vi "CreatePm.vi"(0 "PM_Group in":refnum<class "PM_Group.lvclass">, 5 "error in (no error)":errorcluster, 7 "FPGA API":refnum<class "FPGA API.lvclass">, 9 "ConfigInterface":refnum<class "ConfigInterface.lvclass">, 11 "SV_Publisher":refnum<class "SV_Publisher.lvclass">, 12 "Tags":T1, 13 "Logger":refnum<class "Logger.lvclass">) -> (14 "PM_Group out":refnum<class "PM_Group.lvclass">, 19 "error out":errorcluster)   [LabVIEW 2019, in "PM_Group.lvclass"]
uses:
  PM_Group.lvclass
  C:/Users/H4001/Documents/GitHub/H4000/src/Device_class/Device.lvclass
  C:/Users/H4001/Documents/GitHub/H4000/src/Proccess_class/Proccess.lvclass
  Proccess_class/TAGs.ctl
  FPGA_API_class/FPGA API.lvclass
  ConfigInterface_class/ConfigInterface.lvclass
  SV_Puplisher_class/SV_Publisher.lvclass
  Logger_class/Logger.lvclass
  TypeDef/State PMG.ctl
  PM_Group.lvclass/PM_Group.ctl
  Engine_1DO_2DI_class/DIO.ctl
  FPGA/TypeDef/DO index.ctl
  FPGA/TypeDef/DI index.ctl
  Proccess_class/Proccess.lvclass/Proccess.ctl
  Device_class/Device.lvclass/Device.ctl
  Device_class/Device.lvclass
  Proccess_class/Proccess.lvclass
  Engine_1DO_2DI_class/Engine_1DO_2DI.lvclass
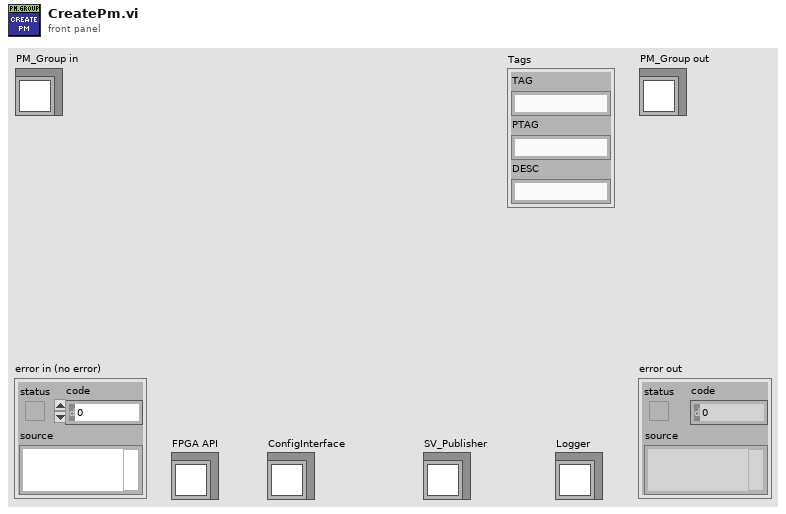
[diagram p1: front panel]
types:
  T1 = typedef "Proccess.lvclass/TAGs.ctl" = cluster{"TAG":string, "PTAG":string, "DESC":string}
  T2 = typedef "State PMG.ctl" = enum16{"NOT READY", "IDLE", "ACTIVE", "ERROR"}
  T3 = typedef "Engine_1DO_2DI.lvclass/DIO.ctl" = cluster{"DO":T4, "DI A":T5, "DI C":T5}
  T4 = typedef "DO index.ctl" = u8
  T5 = typedef "DI index.ctl" = u8
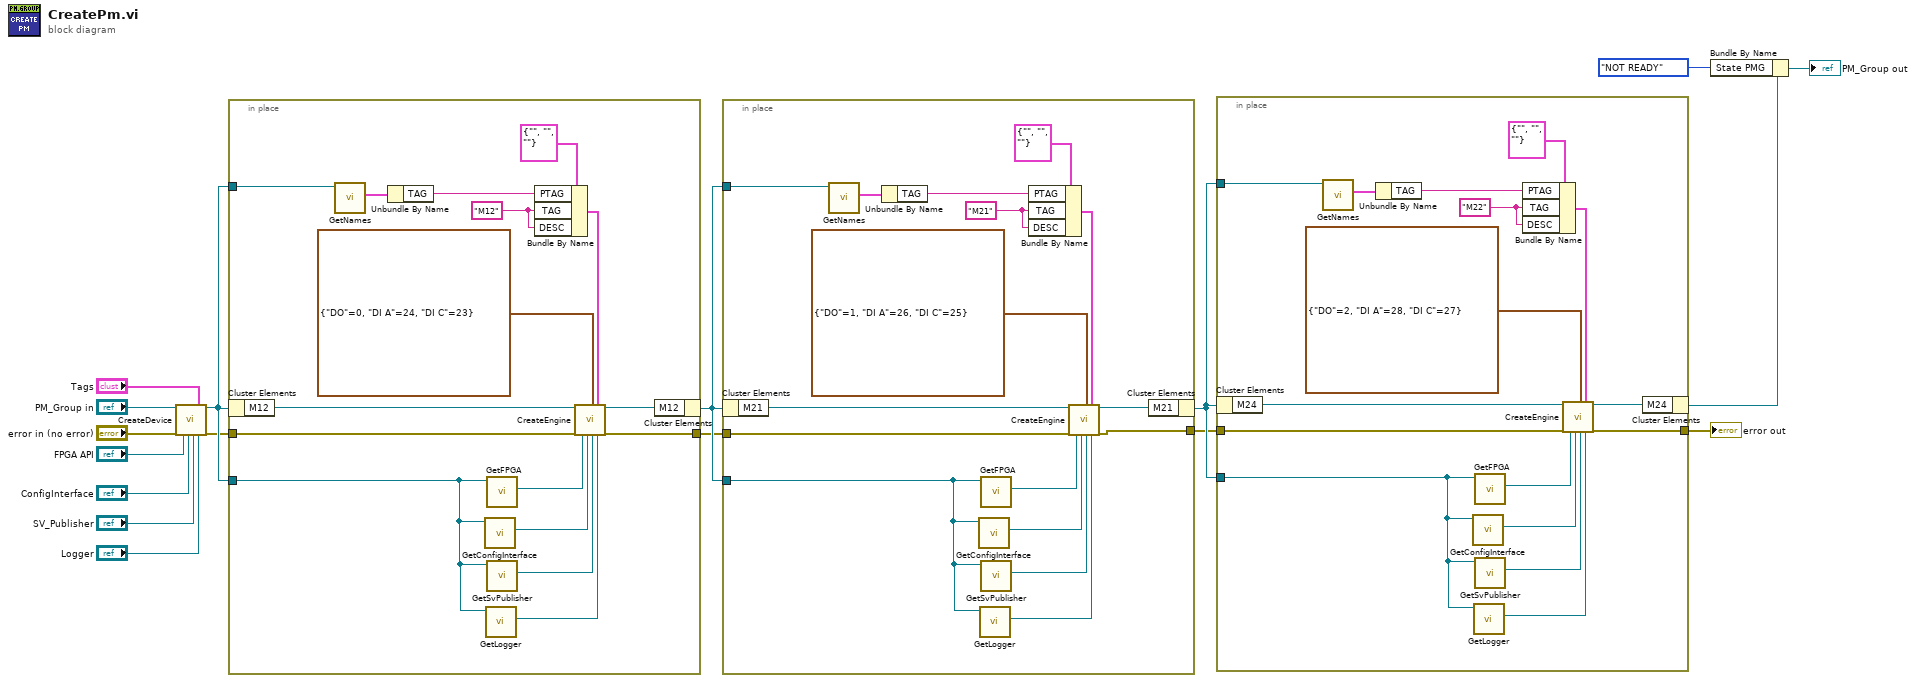
[diagram p0: block diagram]
diagram:
  n1 = call "CreateDevice.vi"("Device in"="PM_Group in", "error in (no error)"="error in (no error)", "FPGA API"="FPGA API", "ConfigInterface"="ConfigInterface", "SV_Publisher"="SV_Publisher", "Tags"="Tags", "Logger"="Logger") -> ("Device out"=w10:refnum<class "PM_Group.lvclass">, "error out"=w9:errorcluster)  [unwired: 11 in]
  n2 = in-place {
    in-place-border: w10 -> [w30]
    in-place-border: w10 -> [w21]
    in-place-border: w9 -> [w19]
    in-place-border: [w18] -> w7
    w25 = "M12" ("TAG")
    n3 = in-place-cluster #1(w10) -> ("M12"=w32:refnum<class "Engine_1DO_2DI.lvclass">)
    n4 = call "GetNames.vi"("Proccess in"=w30) -> ("Tags"=w27:T1)  [unwired: 10 in]
    n5 = Unbundle By Name(w27) -> ("TAG"=w26:string)
    n6 = call "GetConfigInterface.vi"("Device in"=w21) -> ("ConfigInterface"=w22:refnum<class "ConfigInterface.lvclass">)  [unwired: 10 in]
    n7 = call "GetLogger.vi"("Proccess in"=w21) -> ("Logger"=w20:refnum<class "Logger.lvclass">)  [unwired: 10 in]
    n8 = call "GetFPGA.vi"("Device in"=w21) -> ("FPGA API.lvclass"=w24:refnum<class "FPGA API.lvclass">)  [unwired: 10 in]
    n9 = call "GetSvPublisher.vi"("Device in"=w21) -> ("SV_Publisher.lvclass"=w23:refnum<class "SV_Publisher.lvclass">)  [unwired: 10 in]
    n10 = Bundle By Name(cluster=T1 {"TAG"="", "PTAG"="", "DESC"=""} ("Tags"), "PTAG"=w26, "TAG"=w25, "DESC"=w25) -> (w28:T1)
    n11 = call "CreateEngine.vi"("Engine_1DO_2DI in"=w32, "error in (no error)"=w19, "FPGA API"=w24, "ConfigInterface"=w22, "DIO"=T3 {"DO"=0, "DI A"=24, "DI C"=23}, "SV_Publisher"=w23, "Tags"=w28, "Logger"=w20) -> ("Engine_1DO_2DI out"=w31:refnum<class "Engine_1DO_2DI.lvclass">, "error out"=w18:errorcluster)  [unwired: 10 in]
    n12 = in-place-cluster #1("M12"=w31) -> (w8:refnum<class "PM_Group.lvclass">)
  }
  n13 = in-place {
    in-place-border: w8 -> [w46]
    in-place-border: w8 -> [w37]
    in-place-border: w7 -> [w35]
    in-place-border: [w34] -> w5
    w41 = "M21" ("TAG")
    n14 = in-place-cluster #2(w8) -> ("M21"=w48:refnum<class "Engine_1DO_2DI.lvclass">)
    n15 = call "GetNames.vi"("Proccess in"=w46) -> ("Tags"=w43:T1)  [unwired: 10 in]
    n16 = Unbundle By Name(w43) -> ("TAG"=w42:string)
    n17 = call "GetConfigInterface.vi"("Device in"=w37) -> ("ConfigInterface"=w38:refnum<class "ConfigInterface.lvclass">)  [unwired: 10 in]
    n18 = call "GetLogger.vi"("Proccess in"=w37) -> ("Logger"=w36:refnum<class "Logger.lvclass">)  [unwired: 10 in]
    n19 = call "GetFPGA.vi"("Device in"=w37) -> ("FPGA API.lvclass"=w40:refnum<class "FPGA API.lvclass">)  [unwired: 10 in]
    n20 = call "GetSvPublisher.vi"("Device in"=w37) -> ("SV_Publisher.lvclass"=w39:refnum<class "SV_Publisher.lvclass">)  [unwired: 10 in]
    n21 = Bundle By Name(cluster=T1 {"TAG"="", "PTAG"="", "DESC"=""} ("Tags"), "PTAG"=w42, "TAG"=w41, "DESC"=w41) -> (w44:T1)
    n22 = call "CreateEngine.vi"("Engine_1DO_2DI in"=w48, "error in (no error)"=w35, "FPGA API"=w40, "ConfigInterface"=w38, "DIO"=T3 {"DO"=1, "DI A"=26, "DI C"=25}, "SV_Publisher"=w39, "Tags"=w44, "Logger"=w36) -> ("Engine_1DO_2DI out"=w47:refnum<class "Engine_1DO_2DI.lvclass">, "error out"=w34:errorcluster)  [unwired: 10 in]
    n23 = in-place-cluster #2("M21"=w47) -> (w6:refnum<class "PM_Group.lvclass">)
  }
  n24 = in-place {
    in-place-border: w6 -> [w62]
    in-place-border: w6 -> [w53]
    in-place-border: w5 -> [w51]
    in-place-border: [w50] -> w3
    w57 = "M22" ("TAG")
    n25 = in-place-cluster #3(w6) -> ("M24"=w64:refnum<class "Engine_1DO_2DI.lvclass">)
    n26 = call "GetNames.vi"("Proccess in"=w62) -> ("Tags"=w59:T1)  [unwired: 10 in]
    n27 = Unbundle By Name(w59) -> ("TAG"=w58:string)
    n28 = call "GetConfigInterface.vi"("Device in"=w53) -> ("ConfigInterface"=w54:refnum<class "ConfigInterface.lvclass">)  [unwired: 10 in]
    n29 = call "GetLogger.vi"("Proccess in"=w53) -> ("Logger"=w52:refnum<class "Logger.lvclass">)  [unwired: 10 in]
    n30 = call "GetFPGA.vi"("Device in"=w53) -> ("FPGA API.lvclass"=w56:refnum<class "FPGA API.lvclass">)  [unwired: 10 in]
    n31 = call "GetSvPublisher.vi"("Device in"=w53) -> ("SV_Publisher.lvclass"=w55:refnum<class "SV_Publisher.lvclass">)  [unwired: 10 in]
    n32 = Bundle By Name(cluster=T1 {"TAG"="", "PTAG"="", "DESC"=""} ("Tags"), "PTAG"=w58, "TAG"=w57, "DESC"=w57) -> (w60:T1)
    n33 = call "CreateEngine.vi"("Engine_1DO_2DI in"=w64, "error in (no error)"=w51, "FPGA API"=w56, "ConfigInterface"=w54, "DIO"=T3 {"DO"=2, "DI A"=28, "DI C"=27}, "SV_Publisher"=w55, "Tags"=w60, "Logger"=w52) -> ("Engine_1DO_2DI out"=w63:refnum<class "Engine_1DO_2DI.lvclass">, "error out"=w50:errorcluster)  [unwired: 10 in]
    n34 = in-place-cluster #3("M24"=w63) -> (w4:refnum<class "PM_Group.lvclass">)
  }
  "error out" <- w3
  n35 = Bundle By Name(cluster=w4, "State PMG"=State_PMG."NOT READY") -> (→"PM_Group out":refnum<class "PM_Group.lvclass">)
